vi "Collect data from array.vi"() -> ()   [LabVIEW 2021]
panel:
  out "element":dbl
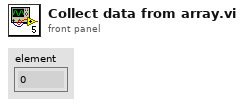
[diagram p1: front panel]
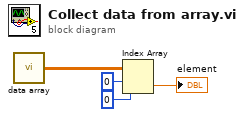
[diagram p0: block diagram]
diagram:
  n1 = call "data array.vi"() -> ("Array"=w4:dbl[][])  [unwired: 11 in]
  n2 = Index Array(array=w4, index (row)=0, index (col)=0 ("disabled index (col)")) -> (element=→"element":dbl)
